vi "Stop.vi"(6 "Busy":refnum<vi>, 8 "error in (no error)":errorcluster, 11 "QuickSilver in":refnum<class "QuickSilver.lvclass">) -> (0 "error out":errorcluster, 2 "String":string, 3 "QuickSilver out":refnum<class "QuickSilver.lvclass">)   [LabVIEW 2018, in "QuickSilver.lvclass"]
uses:
  QuickSilver.lvclass
  QuickSilver.lvclass/QuickSilver.ctl
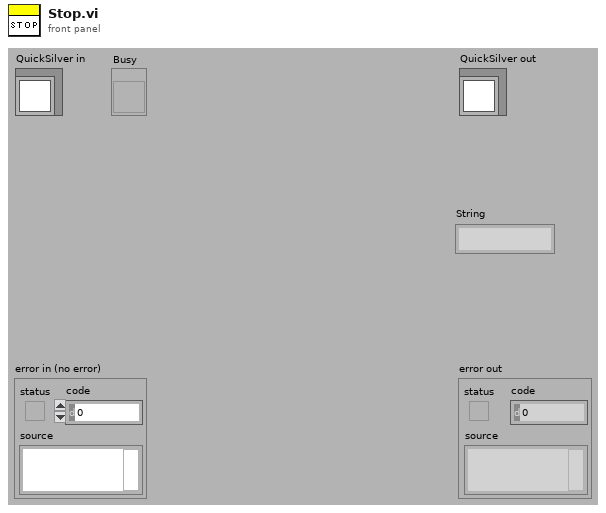
[diagram p1: front panel]
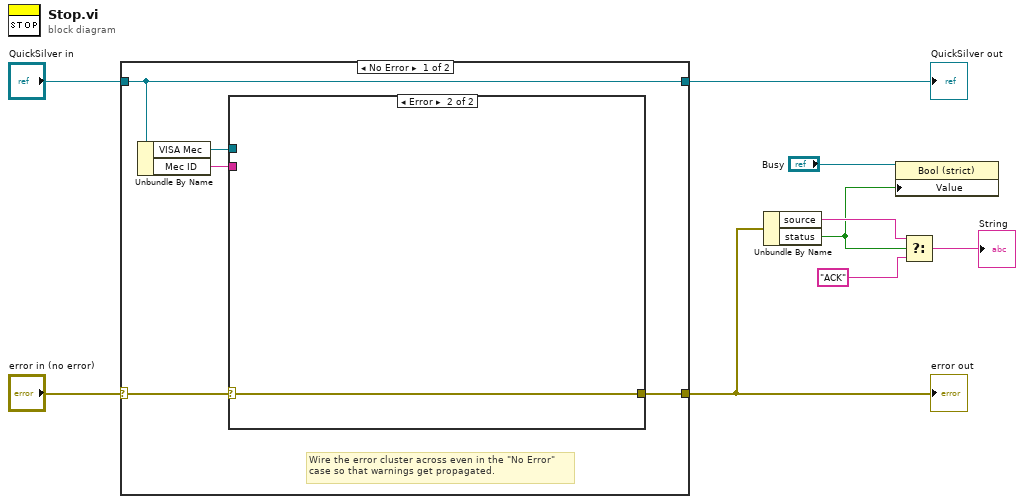
[diagram p0: block diagram]
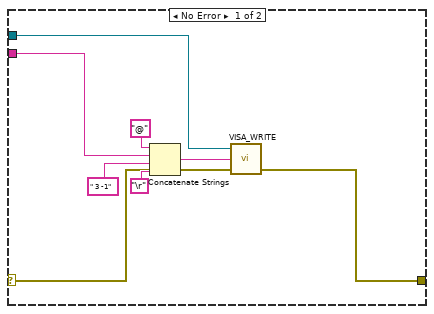
[diagram p2: hidden frame]
diagram:
  n1 = case shown="No Error" "error in (no error)" {
    selector: "error in (no error)" -> [w12 w24]
    tunnel: [w14 w24] -> w4
    tunnel: [w13 w25] -> w8
    tunnel: "QuickSilver in" -> [w13 w25]
    frame No Error {
      # "Wire the error cluster across even in the \"No Error\"\ncase so that warnings get propagated."
      n2 = Unbundle By Name(w13) -> ("VISA Mec"=w11:refnum<visa-resource-name>, "Mec ID"=w10:string)
      n3 = case shown="Error" w12 {
        selector: w12 -> [w16 w23]
        tunnel: [w15 w23] -> w14
        tunnel: w11 -> [w18 _]
        tunnel: w10 -> [w17 _]
        frame No Error {
          n4 = Concatenate Strings("@", w17, " 3 -1", "\r") -> (w19:string)
          n5 = call "VISA_WRITE.vi"("error in (no error)"=w16, "write buffer"=w19, "VISA resource name"=w18) -> ("error out"=w15:errorcluster)  [unwired: 2 out]
        }
        frame Error {
        }
      }
    }
    frame Error {
    }
  }
  "error out" <- w4
  "QuickSilver out" <- w8
  n6 = Unbundle By Name(w4) -> ("source"=w5:string, "status"=w1:bool)
  n7 = property class="Bool (strict)"(reference="Busy", "Value"=w1) -> ()  [unwired: 1 in, 2 out]
  n8 = Select(t=w5, s=w1, f="ACK" ("string")) -> (s? t:f=→"String":string)
